vi "Process Records.vi"(4 "map":T1, 5 "RT hardware channel data":T2[](array[typedef])=[{"channel #"=0, "channel handle"=0, "labels settings for RT"=[]}] {"labels settings for RT"."Label Timestamp Channel Data Reference" format="%.0x"; "labels settings for RT"."Word Initial Raw Value" format="%032.0f"; "labels settings for RT"."Label Disable/Trigger Channel Reference" format="%.0x"; "labels settings for RT"."parameter driver data"."Tx parameter refs" format="%.0x"; "labels settings for RT"."parameter driver data"."Rx block data refs"."Data Reference" format="%.0x"; "labels settings for RT"."SDI" format="%02b"; "labels settings for RT"."label" format="%.0o"}, 6 "error in":errorcluster, 8 "records":T12[](array[typedef]) {"type" format="%04x"; "timestamp" format="%08x"; "msgact" format="%04x"; "data" format="%08x"; "timestamph" format="%08x"}, 9 "parameter values in":dbl[](array[numeric])) -> (0 "error out":errorcluster, 3 "parameter values out":dbl[](array[numeric]))   [LabVIEW 2020, in "Ballard ARINC 429 Engine.lvlib" / "Custom Device.lvlib"]
uses:
  Custom Device.lvlib
  ece6b673-d70a-4abd-8fc5-cd5ecd079ce2.vi
  <instrlib>/BTICardLib/Public/Controls/429 Record.ctl
  <instrlib>/BTICardLib/BTICardLV.lvlib
  <vilib>/NI VeriStand/Custom Device API/Data Reference.ctl
  <vilib>/NI VeriStand/Custom Device API/Custom Device API.lvlib
  <vilib>/NI VeriStand/Custom Device API/Block Data Reference.ctl
  <vilib>/NI VeriStand/Custom Device API/Custom Device Item Ref.ctl
  Shared/Label.ctl
  Encoding and Decoding/Encoding.ctl
  Encoding and Decoding/Encoding and Decoding.lvlib
  Shared/Parameter Definition.ctl
  Shared/RT Parameters.ctl
  Shared/Transfer Type.ctl
  Shared/RT Label Settings.ctl
  Shared/RT Hardware Channel Settings.ctl
  Shared/Map of Identifiers to Indexes.ctl
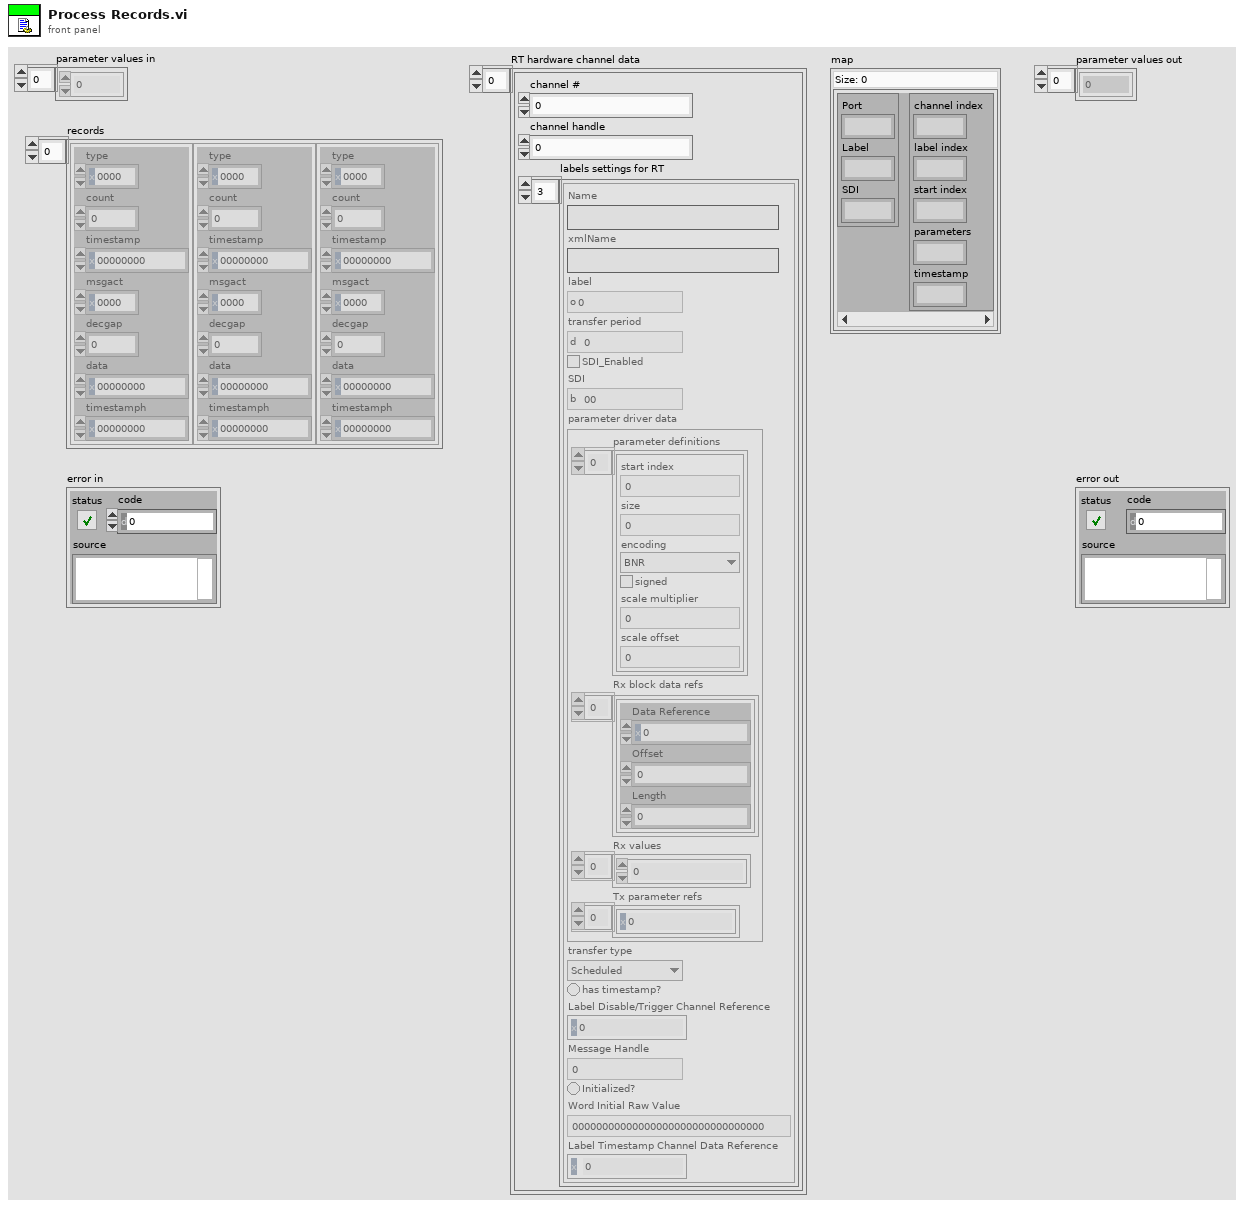
[diagram p1: front panel]
types:
  T1 = typedef "Map of Identifiers to Indexes.ctl" = map{cluster{"Port":u8, "Label":u8, "SDI":u8}, cluster{"channel index":i32, "label index":i32, "start index":i32, "parameters":i32, "timestamp":i32}}
  T2 = typedef "RT Hardware Channel Settings.ctl" = cluster{"channel #":u16, "channel handle":u64, "labels settings for RT":T3[]}
  T3 = typedef "RT Label Settings.ctl" = cluster{"Name":string, "xmlName":string, "label":T4, "transfer period":u32, "SDI_Enabled":bool, "SDI":u8, "parameter driver data":T5, "transfer type":T11, "has timestamp?":bool, "Label Disable/Trigger Channel Reference":T10, "Message Handle":u64, "Initialized?":bool, "Word Initial Raw Value":u32, "Label Timestamp Channel Data Reference":T9}
  T4 = typedef "Label.ctl" = u8
  T5 = typedef "RT Parameters.ctl" = cluster{"parameter definitions":T6[], "Rx block data refs":T8[], "Rx values":dbl[], "Tx parameter refs":T10[]}
  T6 = typedef "Parameter Definition.ctl" = cluster{"start index":i32, "size":i32, "encoding":T7, "signed":bool, "scale multiplier":dbl, "scale offset":dbl}
  T7 = typedef "Encoding and Decoding.lvlib/Encoding.ctl" = enum16{"BNR", "BCD", "Discrete"}
  T8 = typedef "Custom Device API.lvlib/Block Data Reference.ctl" = cluster{"Data Reference":T9, "Offset":u64, "Length":u64}
  T9 = typedef "Custom Device API.lvlib/Data Reference.ctl" = i32
  T10 = typedef "Custom Device API.lvlib/Custom Device Item Ref.ctl" = u64
  T11 = typedef "Transfer Type.ctl" = enum16{"Scheduled", "Acyclic", "Block", "Strobe"}
  T12 = typedef "BTICardLV.lvlib/429 Record.ctl" = cluster{"type":u16, "count":u16, "timestamp":u32, "msgact":u16, "decgap":u16, "data":u32, "timestamph":u32}
  T13 = cluster{"hardware channel":u8, "label":u8, "SDI":u8}
  T14 = cluster{"channel index":i32, "label index":i32, "start index":i32, "parameters":i32, "timestamp":i32}
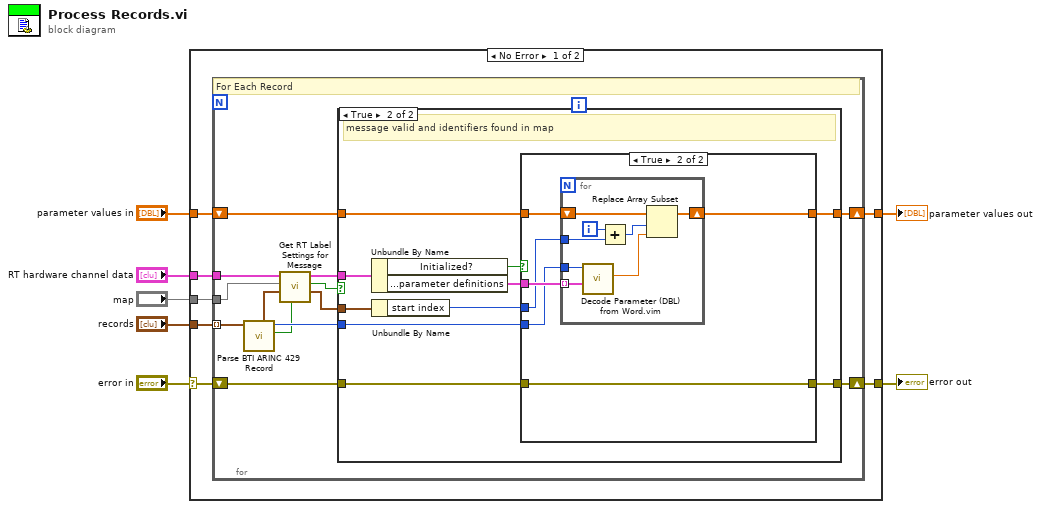
[diagram p0: block diagram]
diagram:
  n1 = case shown="No Error" "error in" {
    selector: "error in" -> [w12 w57]
    tunnel: "records" -> [w11 _]
    tunnel: [w14 w57] -> w6
    tunnel: "RT hardware channel data" -> [w13 _]
    tunnel: [w9 w56] -> w3
    tunnel: "parameter values in" -> [w10 w56]
    tunnel: "map" -> [w8 _]
    frame No Error {
      n2 = for "Process each Record" {
        tunnel: w11 -> [w25] mode=indexing
        shift-right: [w27] -> w14
        shift-left: w12 -> [w26]
        tunnel: w13 -> [w20]
        shift-right: [w22] -> w9
        shift-left: w10 -> [w23]
        tunnel: w8 -> [w17]
        # "For Each Record"
        n3 = call "Parse BTI ARINC 429 Record.vi"("record"=w25) -> ("valid"=w21:bool, "data word"=w24:u32, "message info"=w18:T13)  [unwired: 6 in, 2 out]
        n4 = call "Get RT Label Settings for Message.vi"("valid"=w21, "message identifiers"=w18, "map"=w17, "RT hardware channel data"=w20) -> ("message indexes"=w15:T14, "valid and map exists"=w16:bool, "label settings for RT"=w19:T3)  [unwired: 5 in]
        n5 = case "Channel Found?" shown="True" w16 {
          tunnel: w26 -> [w29 w38]
          tunnel: [w29 w37] -> w27
          tunnel: w24 -> [_ w33]
          tunnel: [w28 w36] -> w22
          tunnel: w23 -> [w28 w34]
          tunnel: w19 -> [_ w32]
          tunnel: w15 -> [_ w31]
          frame False {
            # "message not valid or not found in map"
          }
          frame True {
            # "message valid and identifiers found in map"
            n6 = Unbundle By Name(w32) -> ("Initialized?"=w35:bool, "parameter driver data.parameter definitions"=w39:T6[])
            n7 = Unbundle By Name(w31) -> ("start index"=w30:i32)
            n8 = case shown="True" w35 {
              tunnel: w39 -> [_ w46]
              tunnel: w33 -> [_ w45]
              tunnel: w38 -> [w41 w47]
              tunnel: [w41 w47] -> w37
              tunnel: [w40 w43] -> w36
              tunnel: w34 -> [w40 w44]
              tunnel: w30 -> [_ w42]
              frame False {
                # "This case will be called if users has Labels present on the channel but didn't list them in XML file with \"monitor=false\" in the list.\n\nRecords returned by Read function will have labels (not filtered by HW)."
              }
              frame True {
                n9 = for {
                  tunnel: w46 -> [w55] mode=indexing
                  tunnel: w45 -> [w54]
                  tunnel: w42 -> [w49]
                  shift-right: [w51] -> w43
                  shift-left: w44 -> [w53]
                  i -> [w50]
                  n10 = call "Decode Parameter (DBL) from Word.vim"("parameter definition"=w55, "32-bit word in"=w54) -> ("parameter value"=w52:dbl)  [unwired: 7 in, 2 out]
                  n11 = Add(x=w50, y=w49) -> (x+y=w48:i32)
                  n12 = Replace Array Subset(array=w53, new element=w52, index=w48) -> (w51:dbl[])
                }
              }
            }
          }
        }
      }
    }
    frame Error {
    }
  }
  "error out" <- w6
  "parameter values out" <- w3
